vi "TimerTest.vi"() -> ()   [LabVIEW 2016]
uses:
  main/apis/Setup/GetVI/GetVIByPath.vi
  main/apis/Stimulus/ValueSignal/ValueSignalByPathString.vi
  main/apis/Assert/AssertControlValue/AlmostEqual.vi
  main/Drona.lvlib
  main/apis/Setup/GetVI/GetVI.lvlib
  <vilib>/addons/_JKI Toolkits/Caraya/classes/Test/Test.lvclass
  main/apis/Stimulus/ValueSignal/ValueSignal.lvlib
  main/apis/Assert/AssertControlValue/AssertControlValue.lvlib
panel:
  out "error out":errorcluster
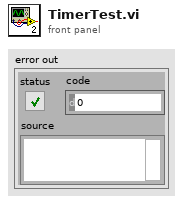
[diagram p1: front panel]
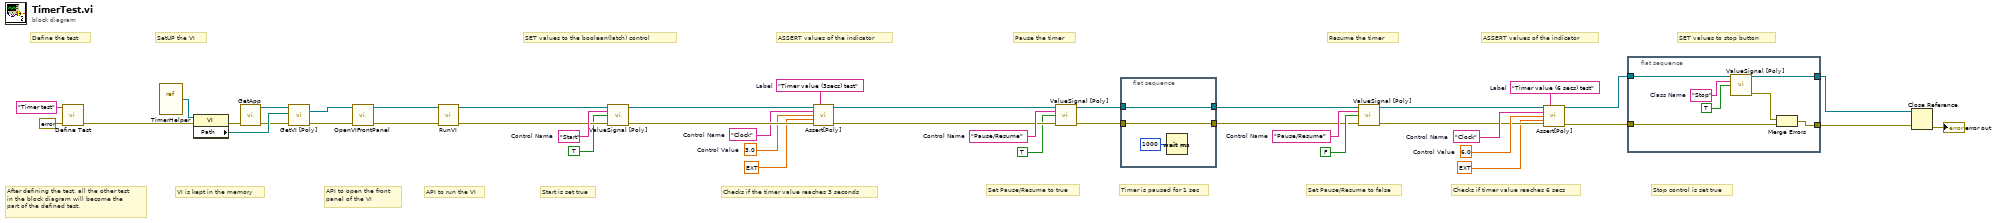
[diagram p0: block diagram]
diagram:
  w8 = "Pause/Resume"  # Control Name
  w17 = "Clock"  # Control Name
  w18 = "Timer value (6 secs) test"  # Label
  w19 = 6.0  # Control Value
  w27 = "Pause/Resume"  # Control Name
  w30 = "Clock"  # Control Name
  w33 = "Timer value (3secs) test"  # Label
  w34 = 3.0  # Control Value
  w32 = "Start"  # Control Name
  # "Resume the timer"
  # "Set Pause/Resume to false"
  # "Timer is paused for 1 sec"
  # "Checks if timer value reaches 6 secs"
  # "ASSERT values of the indicator"
  # "API to open the front\npanel of the VI"
  # "Stop control is set true"
  # "SET values to stop button"
  # "Set Pause/Resume to true"
  # "Pause the timer"
  # "Checks if the timer value reaches 3 seconds"
  # "ASSERT values of the indicator"
  # "Start is set true"
  # "API to run the VI"
  # "SET values to the boolean(latch) control"
  # "VI is kept in the memory"
  # "SetUP the VI"
  # "After defining the test, all the other test\nin the block diagram will become the \npart of the defined test."
  # "Define the test"
  n1 = call <vilib>:"Define Test.vi"("error in (no error)"=errorcluster {"status"=FALSE, "code"=0, "source"=""}, "Label (VI Title)"="Timer test") -> ("error out"=w38:errorcluster)  [unwired: 9 in]
  n2 = vi-ref "TimerHelper.vi"() -> (w31:refnum<vi>)
  n3 = property on="Property Node" class="VI"(reference=w31, error in=w38) -> (error out=w42:errorcluster, "Path"=w41:path)  [unwired: 1 out]
  n4 = call "GetApp.vi"("error in (no error)"=w42) -> ("Application Ref"=w43:refnum<vi>, "error out"=w40:errorcluster)  [unwired: 13 in]
  n5 = call-poly "GetVI [Poly].vi"("Application Ref in"=w43, "VI Path"=w41, "error in (no error)"=w40) -> ("VI Reference"=w21:refnum<vi>, "error out"=w23:errorcluster)  [unwired: 10 in, 1 out]
  n6 = call "OpenVIFrontPanel.vi"("VI Reference In"=w21, "error in"=w23) -> ("VI Reference Out"=w20:refnum<vi>, "error out"=w22:errorcluster)  [unwired: 12 in]
  n7 = call "RunVI.vi"("VI Reference In"=w20, "error in"=w22) -> ("VI Reference Out"=w29:refnum<vi>, "error out"=w28:errorcluster)  [unwired: 12 in]
  n8 = call-poly "ValueSignal [Poly].vi"("VI Reference In"=w29, "Control Path"=w32, "Value (Signaling)"=TRUE, "error in"=w28) -> ("VI Reference Out"=w35:refnum<vi>, "error out"=w36:errorcluster)  [unwired: 10 in]
  n9 = call-poly "Assert[Poly].vi"("VI Reference In"=w35, "Label"=w33, "Control Path"=w30, "Control Value"=w34, "Tolerance"=ext 0.2, "Error In"=w36) -> ("VI Reference Out"=w25:refnum<vi>, "Error Out"=w26:errorcluster)  [unwired: 8 in]
  n10 = call-poly "ValueSignal [Poly].vi"("VI Reference In"=w25, "Control Path"=w27, "Value (Signaling)"=TRUE, "error in"=w26) -> ("VI Reference Out"=w10:refnum<vi>, "error out"=w11:errorcluster)  [unwired: 10 in]
  n11 = flat-sequence {
    tunnel: w11 -> [w45]
    tunnel: [w45] -> w6
    tunnel: w10 -> [w44]
    tunnel: [w44] -> w7
    frame #0 {
      n12 = Wait (ms)(milliseconds to wait=u32 1000) -> ()  [unwired: 1 out]
    }
  }
  n13 = call-poly "ValueSignal [Poly].vi"("VI Reference In"=w7, "Control Path"=w8, "Value (Signaling)"=FALSE, "error in"=w6) -> ("VI Reference Out"=w4:refnum<vi>, "error out"=w5:errorcluster)  [unwired: 10 in]
  n14 = call-poly "Assert[Poly].vi"("VI Reference In"=w4, "Label"=w18, "Control Path"=w17, "Control Value"=w19, "Tolerance"=ext 0.2, "Error In"=w5) -> ("VI Reference Out"=w15:refnum<vi>, "Error Out"=w16:errorcluster)  [unwired: 8 in]
  n15 = flat-sequence {
    tunnel: [w50] -> w1
    tunnel: [w51] -> w2
    tunnel: w15 -> [w49]
    tunnel: w16 -> [w47]
    frame #0 {
      w53 = "Stop"  # Class Name
      n16 = call-poly "ValueSignal [Poly].vi"("VI Reference In"=w49, "Control Path"=w53, "Value (Signaling)"=TRUE) -> ("VI Reference Out"=w51:refnum<vi>, "error out"=w48:errorcluster)  [unwired: 11 in]
      n17 = Merge Errors(w48, w47) -> (w50:errorcluster)
    }
  }
  n18 = Close Reference(reference=w2, error in (no error)=w1) -> (error out=→"error out":errorcluster)
